vi "checkFinishIndirectEnemyPlay.vi"(8 "error in (no error)":errorcluster, 10 "Game":refnum<class "Game.lvclass">, 11 "IndirectEnemyPlay in":refnum<class "IndirectEnemyPlay.lvclass">) -> (0 "error out":errorcluster, 2 "Boolean":bool, 3 "IndirectEnemyPlay out":refnum<class "IndirectEnemyPlay.lvclass">)   [LabVIEW 2020, in "IndirectEnemyPlay.lvclass"]
uses:
  IndirectEnemyPlay.lvclass
  Game_class/Game.lvclass
  Referee_class/command_interpreted.ctl
  Game_class/Game.lvclass/Game.ctl
  Referee_class/Referee.lvclass/Referee.ctl
  Events_class/Events.lvclass/Events.ctl
  Game_class/Read Referee.vi
  Game_class/Read EventsRef.vi
  Events_class/Read ball_out.vi
  Events_class/Read kick.vi
  Referee_class/Read command_interpreted.vi
  Referee_class/Referee.lvclass
  Events_class/Events.lvclass
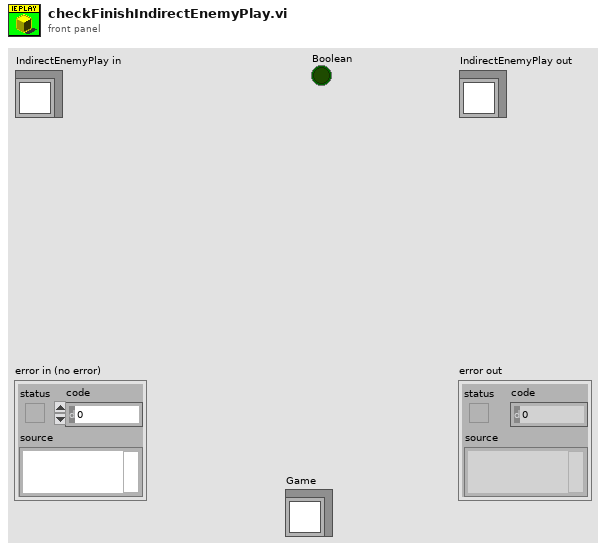
[diagram p1: front panel]
types:
  T1 = typedef "command_interpreted.ctl" = enum16{"Goal Ally", "Goal Enemy", "Ball Placement Enemy", "Ball Placement Ally", "Normal Half Time", "Extra Time  Break", "Extra Half Time", "None", "Post Game", "PKA Normal Start", "Prepare Kickoff Ally", "PKE Normal Start", "Prepare Kickoff Enemy", "Force Start", "Halt", "Timeout", "Prepare Penalty Ally", "Prepare Penalty Enemy", "PPA NormalStart", "PPE Normal Start", "Indirect Free Ally", "Direct Free Enemy", "Direct Free Ally", "Indirect Free Enemy", "Stop"}
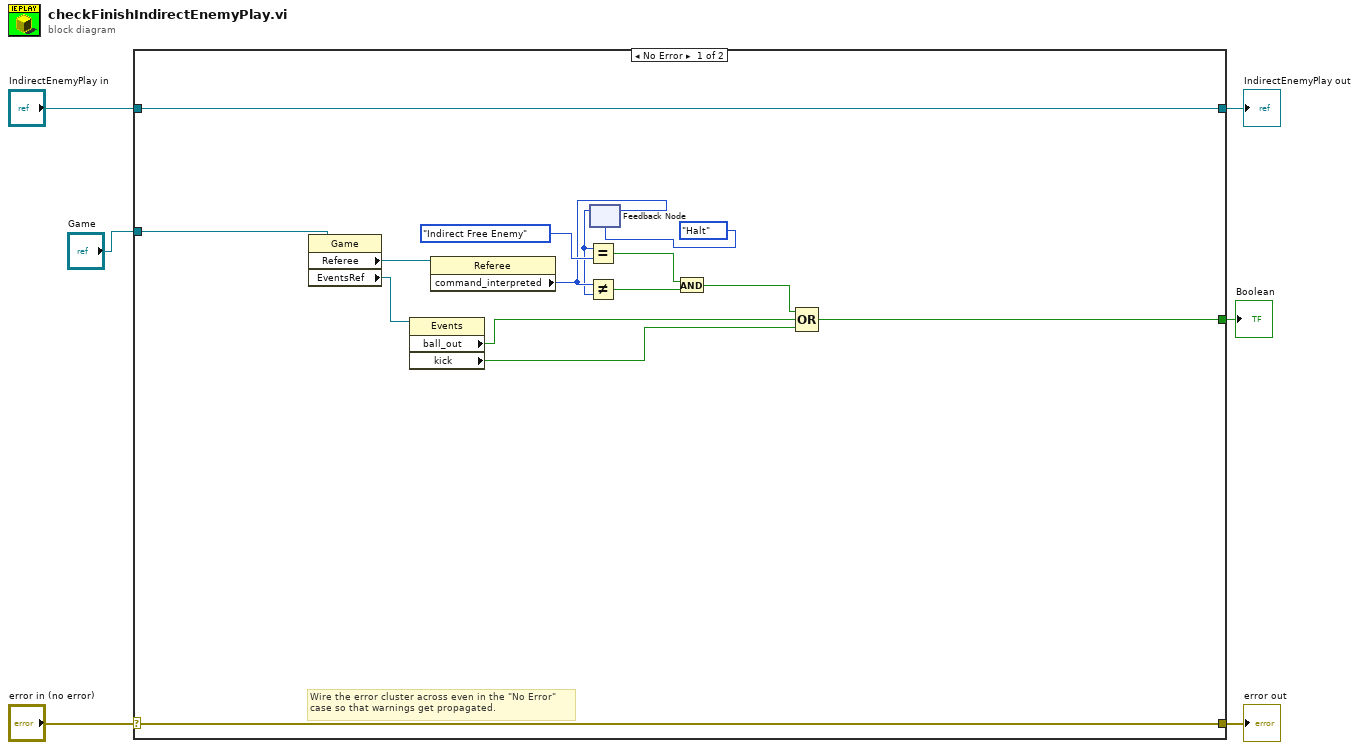
[diagram p0: block diagram]
diagram:
  n1 = case shown="No Error" "error in (no error)" {
    selector: "error in (no error)" -> [w20 w23]
    tunnel: [w20 w23] -> w5
    tunnel: [w21 w22] -> w3
    tunnel: "IndirectEnemyPlay in" -> [w21 w22]
    tunnel: "Game" -> [w9 _]
    tunnel: [w8 _] -> w1
    frame No Error {
      # "Wire the error cluster across even in the \"No Error\"\ncase so that warnings get propagated."
      n2 = property class="Game"(reference=w9) -> ("Referee"=w19:refnum<class "Referee.lvclass">, "EventsRef"=w12:refnum<class "Events.lvclass">)  [unwired: 1 in, 2 out]
      n3 = property class="Events"(reference=w12) -> ("ball_out"=w10:bool, "kick"=w7:bool)  [unwired: 1 in, 2 out]
      n4 = property class="Referee"(reference=w19) -> ("command_interpreted"=w16:T1)  [unwired: 1 in, 2 out]
      n5 = feedback #1(command_interpreted."Halt" ("command_interpreted")) -> (w15:T1)
      n6 = Equal?(x=w15, y=command_interpreted."Indirect Free Enemy" ("command_interpreted")) -> (x = y?=w17:bool)
      n7 = Not Equal?(x=w16, y=w15) -> (x != y?=w14:bool)
      n8 = feedback-in #1(w16) -> ()
      n9 = And(x=w17, y=w14) -> (x .and. y?=w11:bool)
      n10 = Compound Arithmetic op=OR(w11, w10, w7) -> (w8:bool)
    }
    frame Error {
    }
  }
  "error out" <- w5
  "IndirectEnemyPlay out" <- w3
  "Boolean" <- w1
